vi "pH clear.vi"(3 "index":i32) -> (1 "Buffers":T1(array[cluster]) {"V/T" format="%.2f"; "Buffer" format="%.2f"})   [LabVIEW 2012]
uses:
  global scale array.vi
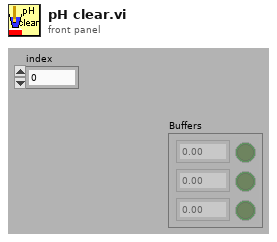
[diagram p1: front panel]
types:
  T1 = cluster{"Buffer":dbl, "Calibrated":bool, "V/T":dbl}[]
  T2 = typedef "calib array.ctl" = T3[]
  T3 = typedef "conversion.ctl" = cluster{"conversion matrix":sgl[][], "units":string, "name":string, "scale type":T4, "offset (volts)":dbl, "second channel":i8, "correspondence table":T5, "offset (physical units)":dbl, "pH scale":T6, "D.O.":T7}
  T4 = typedef "scale type.ctl" = enum16{"Volts", "Polynomial", "Correspondence Table", "pH", "Dissolved Oxygen", "Quadratic"}
  T5 = typedef "correspondence table.ctl" = cluster{"physical units":dbl, "volts":dbl}[]
  T6 = typedef "pH scale.ctl" = cluster{"Buffers":cluster{"Buffer":dbl, "Calibrated":bool, "V/T":dbl}[], "Temperature":dbl}
  T7 = typedef "DO scale.ctl" = cluster{"Temperature":dbl, "K":dbl, "barometric pressure":dbl}
  T8 = cluster{"Buffer":dbl, "Calibrated":bool, "V/T":dbl}
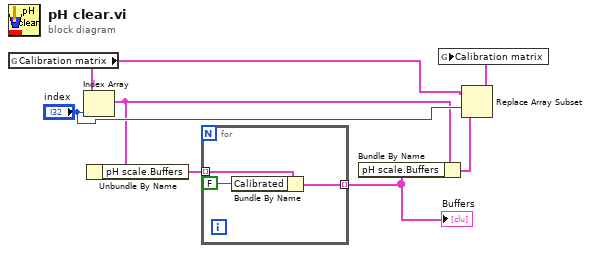
[diagram p0: block diagram]
diagram:
  n1 = global read "global scale array.vi" "Calibration matrix"() -> (w7:T2)
  n2 = Index Array(array=w7, index="index") -> (element=w3:T3)
  n3 = Unbundle By Name(w3) -> ("pH scale.Buffers"=w2:T1)
  n4 = for {
    tunnel: w2 -> [w10] mode=indexing
    tunnel: [w9] -> w1 mode=indexing
    n5 = Bundle By Name(cluster=w10, "Calibrated"=FALSE) -> (w9:T8)
  }
  "Buffers" <- w1
  n6 = Bundle By Name(cluster=w3, "pH scale.Buffers"=w1) -> (w6:T3)
  n7 = Replace Array Subset(array=w7, new element=w6, index="index") -> (w4:T2)
  n8 = global write "global scale array.vi" "Calibration matrix"(w4) -> ()
